vi "log analysis_gps.vi"() -> ()   [LabVIEW 2018] (continued)
-0.105000\n\t\n15:09:27.3\tlog_raw\tgps_raw\t#INSPVAXA,USB3,0,49.0,FINESTEERING,2107,281385.350,02000000,471d,15824;INS_ALIGNMENT_COMPLETE,INS_RTKFIXED,37.37092984687,126.72160192884,8.2009,22.3000,0.3659,0.2906,-0.0108,-0.966416737,-0.773960288,33.451430049,0.4185,0.2991,0.5729,0.1134,0.0948,0.0848,0.2660,0.2403,5.1498,0f000001,0*c2089fa9\n\tsystem status\tnormal 2 28.200000 0 0\trobot status\t67.923992\t88.748599\t8.200900\t-0.966417\t-0.773960\t56.548570\t0.472000\t0.029000\n\t\n15:09:27.8\tlog_raw\tgps_raw\t#INSPVAXA,USB3,0,49.0,FINESTEERING,2107,281385.850,02000000,471d,15824;INS_ALIGNMENT_COMPLETE,INS_RTKFIXED,37.37093156972,126.72160349245,8.1991,22.3000,0.3552,0.2819,0.0017,-0.982402524,-0.987093830,33.457221519,0.4185,0.2991,0.5729,0.1134,0.0948,0.0848,0.2660,0.2403,5.1498,0f000001,0*8db597c9\n\tsystem status\tnormal 2 28.200000 0 0\trobot status\t68.062494\t88.939808\t8.199100\t-0.982403\t-0.987094\t56.542778\t0.454000\t0.050000\n\t\n15:09:28.3\tlog_raw\tgps_raw\t\tsystem status\tnormal 2 28.200000 0 0\trobot status\t68.185778\t89.112120\t8.198400\t-0.951225\t-0.966912\t56.644351\t0.454000\t0.068000\n\t\n15:09:28.8\tlog_raw\tgps_raw\t#INSPVAXA,USB3,0,46.0,FINESTEERING,2107,281386.850,02000000,471d,15824;INS_ALIGNMENT_COMPLETE,INS_RTKFIXED,37.37093500656,126.72160657159,8.1978,22.3000,0.3860,0.2986,-0.0065,-0.930872832,-0.693352418,33.361120344,0.4182,0.2979,0.5715,0.1134,0.0948,0.0846,0.2660,0.2403,5.1494,0f000001,0*a8ec127a\n\tsystem status\tnormal 2 28.200000 0 0\trobot status\t68.335239\t89.321242\t8.197800\t-0.930873\t-0.693352\t56.638880\t0.495000\t0.011000\n\t\n15:09:29.3\tlog_raw\tgps_raw\t\tsystem status\tnormal 2 28.200000 0 0\trobot status\t68.463353\t89.496075\t8.196000\t-0.864589\t-0.927789\t56.656049\t0.556000\t-0.113000\n\t\n15:09:29.8\tlog_raw\tgps_raw\t#INSPVAXA,USB3,0,48.5,FINESTEERING,2107,281387.850,02000000,471d,15824;INS_ALIGNMENT_COMPLETE,INS_RTKFIXED,37.37093847805,126.72160977606,8.1934,22.3000,0.3545,0.2733,-0.0290,-0.871913936,-1.019858036,33.407520693,0.4181,0.2974,0.5707,0.1132,0.0948,0.0844,0.2660,0.2403,5.1492,0f000001,0*8b26d1b5\n\tsystem status\tnormal 2 28.200000 0 0\trobot status\t68.619086\t89.706522\t8.193400\t-0.871914\t-1.019858\t56.592479\t0.417000\t0.094000\n\t\n15:09:30.3\tlog_raw\tgps_raw\t\tsystem status\tnormal 2 28.200000 0 0\trobot status\t68.741379\t89.875198\t8.191600\t-0.846087\t-0.843708\t56.650263\t0.529000\t-0.019000\n\t\n15:09:30.8\tlog_raw\tgps_raw\t#INSPVAXA,USB3,0,47.0,FINESTEERING,2107,281388.850,02000000,471d,15824;INS_ALIGNMENT_COMPLETE,INS_RTKFIXED,37.37094185798,126.72161284652,8.1862,22.3000,0.3458,0.2807,0.0000,-0.647146834,-0.755815505,33.229882391,0.4177,0.2968,0.5693,0.1134,0.0951,0.0842,0.2659,0.2403,5.1493,0f000001,0*e04b9d7e\n\tsystem status\tnormal 2 28.200000 0 0\trobot status\t68.891062\t90.081640\t8.186200\t-0.647147\t-0.755816\t56.770118\t0.433000\t0.079000\n\t\n15:09:31.3\tlog_raw\tgps_raw\t\tsystem status\tnormal 2 28.200000 0 0\trobot status\t69.018551\t90.258982\t8.184300\t-0.770006\t-0.647307\t56.616583\t0.456000\t0.062000\n\t\n15:09:31.8\tlog_raw\tgps_raw\t#INSPVAXA,USB3,0,51.0,FINESTEERING,2107,281389.850,02000000,471d,15824;INS_ALIGNMENT_COMPLETE,INS_RTKFIXED,37.37094531152,126.72161597043,8.1814,22.3000,0.3770,0.3007,-0.0075,-0.964998734,-0.610692019,33.331132112,0.4178,0.2983,0.5697,0.1133,0.0955,0.0841,0.2659,0.2402,5.1491,0f000001,0*f3e7f4f6\n\tsystem status\tnormal 2 28.200000 0 0\trobot status\t69.167773\t90.464927\t8.181400\t-0.964999\t-0.610692\t56.668868\t0.457000\t0.069000\n\t\n15:09:32.3\tlog_raw\tgps_raw\t#INSPVAXA,USB3,0,50.5,FINESTEERING,2107,281390.350,02000000,471d,15824;INS_ALIGNMENT_COMPLETE,INS_RTKFIXED,37.37094699615,126.72161749721,8.1810,22.3000,0.3585,0.2781,-0.0176,-0.963426361,-0.735868518,33.269975778,0.4179,0.2987,0.5691,0.1132,0.0952,0.0837,0.2658,0.2402,5.1481,0f000001,0*d9e47fdc\n\tsystem status\tnormal 2 28.200000 0 0\trobot status\t69.303012\t90.651894\t8.181000\t-0.963426\t-0.735869\t56.730024\t0.431000\t0.076000\n\t\n15:09:32.8\tlog_raw\tgps_raw\t#INSPVAXA,USB3,0,50.5,FINESTEERING,2107,281390.850,02000000,471d,15824;INS_ALIGNMENT_COMPLETE,INS_RTKFIXED,37.37094874032,126.72161908849,8.1805,22.3000,0.3294,0.2293,-0.0009,-0.908401670,-0.595727338,33.364278854,0.4179,0.2987,0.5691,0.1132,0.0952,0.0837,0.2658,0.2402,5.1481,0f000001,0*5999a9d2\n\tsystem status\tnormal 2 28.200000 0 0\trobot status\t69.443965\t90.845469\t8.180500\t-0.908402\t-0.595727\t56.635721\t0.644000\t-0.257000\n\t\n15:09:33.3\tlog_raw\tgps_raw\t#INSPVAXA,USB3,0,48.0,FINESTEERING,2107,281391.350,02000000,471d,15824;INS_ALIGNMENT_COMPLETE,INS_RTKFIXED,37.37095049924,126.72162069173,8.1796,22.3000,0.4034,0.3085,-0.0112,-0.795383493,-0.971346032,33.378242699,0.4182,0.2986,0.5686,0.1132,0.0949,0.0836,0.2658,0.2402,5.1464,0f000001,0*1e48eff8\n\tsystem status\tnormal 2 28.200000 0 0\trobot status\t69.585978\t91.040681\t8.179600\t-0.795383\t-0.971346\t56.621757\t0.521000\t-0.011000\n\t\n15:09:33.8\tlog_raw\tgps_raw\t#INSPVAXA,USB3,0,48.0,FINESTEERING,2107,281391.850,02000000,471d,15824;INS_ALIGNMENT_COMPLETE,INS_RTKFIXED,37.37095218768,126.72162223158,8.1782,22.3000,0.3736,0.3039,0.0085,-0.869440972,-1.042554722,33.323263236,0.4182,0.2986,0.5686,0.1132,0.0949,0.0836,0.2658,0.2402,5.1464,0f000001,0*be662b3c\n\tsystem status\tnormal 2 28.200000 0 0\trobot status\t69.722375\t91.228070\t8.178200\t-0.869441\t-1.042555\t56.676737\t0.524000\t-0.028000\n\t\n15:09:34.3\tlog_raw\tgps_raw\t\tsystem status\tnormal 2 28.200000 0 0\trobot status\t69.851097\t91.401055\t8.175700\t-0.533369\t-1.495352\t56.519855\t0.436000\t0.040000\n\t\n15:09:34.8\tlog_raw\tgps_raw\t#INSPVAXA,USB3,0,46.5,FINESTEERING,2107,281392.850,02000000,471d,15824;INS_ALIGNMENT_COMPLETE,INS_RTKFIXED,37.37095563956,126.72162543709,8.1738,22.3000,0.3750,0.2874,-0.0042,-0.381103782,-1.196591916,33.536451772,0.4182,0.2976,0.5666,0.1131,0.0944,0.0833,0.2657,0.2401,5.1446,0f000001,0*fd2c5164\n\tsystem status\tnormal 2 28.200000 0 0\trobot status\t70.006314\t91.611174\t8.173800\t-0.381104\t-1.196592\t56.463548\t0.516000\t-0.027000\n\t\n15:09:35.3\tlog_raw\tgps_raw\t#INSPVAXA,USB3,0,47.0,FINESTEERING,2107,281393.350,02000000,471d,15824;INS_ALIGNMENT_COMPLETE,INS_RTKFIXED,37.37095732903,126.72162695963,8.1710,22.3000,0.3684,0.2951,-0.0131,-0.615904330,-1.127921907,33.544859726,0.4171,0.2952,0.5633,0.1132,0.0946,0.0833,0.2656,0.2401,5.1445,0f000001,0*dbe231da\n\tsystem status\tnormal 2 28.200000 0 0\trobot status\t70.141178\t91.798678\t8.171000\t-0.615904\t-1.127922\t56.455140\t0.493000\t0.009000\n\t\n15:09:35.8\tlog_raw\tgps_raw\t#INSPVAXA,USB3,0,47.0,FINESTEERING,2107,281393.850,02000000,471d,15824;INS_ALIGNMENT_COMPLETE,INS_RTKFIXED,37.37095908537,126.72162857603,8.1657,22.3000,0.3533,0.2801,-0.0216,-0.431209048,-1.265989093,33.662345403,0.4171,0.2952,0.5633,0.1132,0.0946,0.0833,0.2656,0.2401,5.1445,0f000001,0*22a3a0dc\n\tsystem status\tnormal 2 28.200000 0 0\trobot status\t70.284356\t91.993603\t8.165700\t-0.431209\t-1.265989\t56.337655\t0.473000\t0.013000\n\t\n15:09:36.3\tlog_raw\tgps_raw\t#INSPVAXA,USB3,0,49.5,FINESTEERING,2107,281394.350,02000000,471d,15824;INS_ALIGNMENT_COMPLETE,INS_RTKFIXED,37.37096076368,126.72163015176,8.1608,22.3000,0.3647,0.2816,-0.0115,-0.296506050,-1.118124475,33.712011853,0.4164,0.2937,0.5589,0.1136,0.0946,0.0836,0.2655,0.2400,5.1444,0f000001,0*688a566e\n\tsystem status\tnormal 2 28.200000 0 0\trobot status\t70.423932\t92.179869\t8.160800\t-0.296506\t-1.118124\t56.287988\t0.497000\t0.000000\n\t\n15:09:36.8\tlog_raw\tgps_raw\t#INSPVAXA,USB3,0,49.5,FINESTEERING,2107,281394.850,02000000,471d,15824;INS_ALIGNMENT_COMPLETE,INS_RTKFIXED,37.37096245961,126.72163173093,8.1552,22.3000,0.3611,0.2897,0.0065,-0.395039042,-1.114938757,33.806057490,0.4164,0.2937,0.5589,0.1136,0.0946,0.0836,0.2655,0.2400,5.1444,0f000001,0*207a4651\n\tsystem status\tnormal 2 28.200000 0 0\trobot status\t70.563812\t92.368089\t8.155200\t-0.395039\t-1.114939\t56.193943\t0.482000\t0.013000\n\t\n15:09:37.3\tlog_raw\tgps_raw\t\tsystem status\tnormal 2 28.200000 0 0\trobot status\t70.685779\t92.532461\t8.150200\t-0.328345\t-0.854593\t56.176913\t0.501000\t-0.012000\n\t\n15:09:37.8\tlog_raw\tgps_raw\t#INSPVAXA,USB3,0,47.5,FINESTEERING,2107,281395.850,02000000,471d,15824;INS_ALIGNMENT_COMPLETE,INS_RTKFIXED,37.37096587417,126.72163486610,8.1446,22.3000,0.3698,0.2924,-0.0143,-0.371056293,-0.946940262,33.969984358,0.4152,0.2922,0.5549,0.1139,0.0950,0.0842,0.2655,0.2400,5.1444,0f000001,0*416a3ff6\n\tsystem status\tnormal 2 28.200000 0 0\trobot status\t70.841520\t92.747051\t8.144600\t-0.371056\t-0.946940\t56.030016\t0.509000\t-0.014000\n\t\n15:09:38.3\tlog_raw\tgps_raw\t#INSPVAXA,USB3,0,47.5,FINESTEERING,2107,281396.350,02000000,471d,15824;INS_ALIGNMENT_COMPLETE,INS_RTKFIXED,37.37096753829,126.72163640742,8.1378,22.3000,0.3398,0.2681,-0.0087,-0.164596770,-1.133388969,33.930144164,0.4145,0.2919,0.5524,0.1132,0.0937,0.0831,0.2654,0.2399,5.1441,0f000001,0*c9e3845c\n\tsystem status\tnormal 2 28.200000 0 0\trobot status\t70.978048\t92.931741\t8.137800\t-0.164597\t-1.133389\t56.069856\t0.415000\t0.100000\n\t\n15:09:38.8\tlog_raw\tgps_raw\t#INSPVAXA,USB3,0,47.5,FINESTEERING,2107,281396.850,02000000,471d,15824;INS_ALIGNMENT_COMPLETE,INS_RTKFIXED,37.37096924651,126.72163797428,8.1309,22.3000,0.3574,0.2705,-0.0020,-0.147004218,-0.814443066,33.921255816,0.4145,0.2919,0.5524,0.1132,0.0937,0.0831,0.2654,0.2399,5.1441,0f000001,0*98005433\n\tsystem status\tnormal 2 28.200000 0 0\trobot status\t71.116838\t93.121326\t8.130900\t-0.147004\t-0.814443\t56.078744\t0.431000\t0.089000\n\t\n15:09:39.3\tlog_raw\tgps_raw\t#INSPVAXA,USB3,0,49.5,FINESTEERING,2107,281397.350,02000000,471d,15824;INS_ALIGNMENT_COMPLETE,INS_RTKFIXED,37.37097094637,126.72163952751,8.1230,22.3000,0.3568,0.2763,-0.0303,-0.204424116,-0.677389898,33.930384401,0.4166,0.2976,0.5621,0.1134,0.0950,0.0840,0.2655,0.2398,5.1447,0f000001,0*229e290a\n\tsystem status\tnormal 2 28.200000 0 0\trobot status\t71.254420\t93.309983\t8.123000\t-0.204424\t-0.677390\t56.069616\t0.437000\t0.088000\n\t\n15:09:39.8\tlog_raw\tgps_raw\t#INSPVAXA,USB3,0,49.5,FINESTEERING,2107,281397.850,02000000,471d,15824;INS_ALIGNMENT_COMPLETE,INS_RTKFIXED,37.37097267317,126.72164110503,8.1156,22.3000,0.3644,0.2601,0.0030,-0.207601893,-0.850493393,33.903346021,0.4166,0.2976,0.5621,0.1134,0.0950,0.0840,0.2655,0.2398,5.1447,0f000001,0*99e15a33\n\tsystem status\tnormal 2 28.200000 0 0\trobot status\t71.394154\t93.501630\t8.115600\t-0.207602\t-0.850493\t56.096654\t0.434000\t0.077000\n\t\n15:09:40.3\tlog_raw\tgps_raw\t#INSPVAXA,USB3,0,47.0,FINESTEERING,2107,281398.350,02000000,471d,15824;INS_ALIGNMENT_COMPLETE,INS_RTKFIXED,37.37097438871,126.72164266550,8.1100,22.3000,0.3561,0.2764,-0.0101,-0.236656715,-0.969278432,33.883238770,0.4175,0.2995,0.5669,0.1134,0.0951,0.0842,0.2654,0.2398,5.1455,0f000001,0*71e938c6\n\tsystem status\tnormal 2 28.200000 0 0\trobot status\t71.532378\t93.692028\t8.110000\t-0.236657\t-0.969278\t56.116761\t0.440000\t0.086000\n\t\n15:09:40.8\tlog_raw\tgps_raw\t#INSPVAXA,USB3,0,47.0,FINESTEERING,2107,281398.850,02000000,471d,15824;INS_ALIGNMENT_COMPLETE,INS_RTKFIXED,37.37097610679,126.72164421082,8.1028,22.3000,0.3606,0.2818,-0.0239,-0.382752172,-0.849124601,34.007737280,0.4175,0.2995,0.5669,0.1134,0.0951,0.0842,0.2654,0.2398,5.1455,0f000001,0*8bea9a1b\n\tsystem status\tnormal 2 28.200000 0 0\trobot status\t71.669260\t93.882707\t8.102800\t-0.382752\t-0.849125\t55.992263\t0.544000\t-0.080000\n\t\n15:09:41.3\tlog_raw\tgps_raw\t#INSPVAXA,USB3,0,48.0,FINESTEERING,2107,281399.350,02000000,471d,15824;INS_ALIGNMENT_COMPLETE,INS_RTKFIXED,37.37097781437,126.72164579637,8.0962,22.3000,0.3464,0.2856,-0.0229,-0.220443352,-0.638082090,34.139023670,0.4187,0.3008,0.5721,0.1133,0.0950,0.0843,0.2654,0.2397,5.1467,0f000001,0*4de46431\n\tsystem status\tnormal 2 28.200000 0 0\trobot status\t71.809706\t94.072221\t8.096200\t-0.220443\t-0.638082\t55.860976\t0.490000\t-0.003000\n\t\n15:09:41.8\tlog_raw\tgps_raw\t#INSPVAXA,USB3,0,48.0,FINESTEERING,2107,281399.850,02000000,471d,15824;INS_ALIGNMENT_COMPLETE,INS_RTKFIXED,37.37097954920,126.72164741016,8.0894,22.3000,0.3776,0.2848,-0.0077,-0.220802619,-0.919793940,34.236212275,0.4187,0.3008,0.5721,0.1133,0.0950,0.0843,0.2654,0.2397,5.1467,0f000001,0*1294b3ed\n\tsystem status\tnormal 2 28.200000 0 0\trobot status\t71.952652\t94.264759\t8.089400\t-0.220803\t-0.919794\t55.763788\t0.496000\t-0.003000\n\t\n15:09:42.3\tlog_raw\tgps_raw\t#INSPVAXA,USB3,0,51.0,FINESTEERING,2107,281400.350,02000000,471d,15824;INS_ALIGNMENT_COMPLETE,INS_RTKFIXED,37.37098127121,126.72164900828,8.0835,22.3000,0.3512,0.2798,-0.0167,-0.348314510,-1.071908763,34.359634607,0.4200,0.3034,0.5796,0.1133,0.0952,0.0845,0.2654,0.2397,5.1479,0f000001,0*0d7d68ff\n\tsystem status\tnormal 2 28.200000 0 0\trobot status\t72.094211\t94.455874\t8.083500\t-0.348315\t-1.071909\t55.640365\t0.488000\t0.004000\n\t\n15:09:42.8\tlog_raw\tgps_raw\t\tsystem status\tnormal 2 28.200000 0 0\trobot status\t72.235639\t94.643836\t8.077100\t-0.443262\t-0.875036\t55.562836\t0.488000\t0.000000\n\t\n15:09:43.3\tlog_raw\tgps_raw\t#INSPVAXA,USB3,0,47.5,FINESTEERING,2107,281401.350,02000000,471d,15824;INS_ALIGNMENT_COMPLETE,INS_RTKFIXED,37.37098468255,126.72165224111,8.0693,22.3000,0.3522,0.2654,-0.0166,-0.377347631,-0.696818935,34.675390534,0.4199,0.3031,0.5827,0.1133,0.0950,0.0845,0.2653,0.2397,5.1493,0f000001,0*9d8e74ce\n\tsystem status\tnormal 2 28.200000 0 0\trobot status\t72.380570\t94.834478\t8.069300\t-0.377348\t-0.696819\t55.324609\t0.489000\t-0.012000\n\t\n15:09:43.8\tlog_raw\tgps_raw\t#INSPVAXA,USB3,0,47.5,FINESTEERING,2107,281401.850,02000000,471d,15824;INS_ALIGNMENT_COMPLETE,INS_RTKFIXED,37.37098640066,126.72165387594,8.0604,22.3000,0.3637,0.3053,-0.0327,-0.270135271,-0.804168366,34.795363793,0.4199,0.3031,0.5827,0.1133,0.0950,0.0845,0.2653,0.2397,5.1493,0f000001,0*da64b754\n\tsystem status\tnormal 2 28.200000 0 0\trobot status\t72.525381\t95.025161\t8.060400\t-0.270135\t-0.804168\t55.204636\t0.506000\t-0.006000\n\t\n15:09:44.3\tlog_raw\tgps_raw\t#INSPVAXA,USB3,0,50.5,FINESTEERING,2107,281402.350,02000000,471d,15824;INS_ALIGNMENT_COMPLETE,INS_RTKFIXED,37.37098814311,126.72165553313,8.0529,22.3000,0.3514,0.2761,-0.0227,-0.415994366,-1.222362731,34.800018159,0.4207,0.3056,0.5893,0.1133,0.0953,0.0846,0.2653,0.2396,5.1507,0f000001,0*f3097738\n\tsystem status\tnormal 2 28.200000 0 0\trobot status\t72.672172\t95.218545\t8.052900\t-0.415994\t-1.222363\t55.199982\t0.505000\t-0.016000\n\t\n15:09:44.8\tlog_raw\tgps_raw\t#INSPVAXA,USB3,0,50.5,FINESTEERING,2107,281402.850,02000000,471d,15824;INS_ALIGNMENT_COMPLETE,INS_RTKFIXED,37.37098982425,126.72165714706,8.0452,22.3000,0.3664,0.2820,-0.0237,-0.514294339,-1.108715950,34.873142980,0.4207,0.3056,0.5893,0.1133,0.0953,0.0846,0.2653,0.2396,5.1507,0f000001,0*3533bd5f\n\tsystem status\tnormal 2 28.200000 0 0\trobot status\t72.815131\t95.405124\t8.045200\t-0.514294\t-1.108716\t55.126857\t0.489000\t0.035000\n\t\n15:09:45.3\tlog_raw\tgps_raw\t#INSPVAXA,USB3,0,46.5,FINESTEERING,2107,281403.350,02000000,471d,15824;INS_ALIGNMENT_COMPLETE,INS_RTKFIXED,37.37099150836,126.72165880250,8.0350,22.3000,0.3619,0.2923,-0.0388,-0.135694474,-1.036034406,34.888546976,0.4207,0.3066,0.5937,0.1132,0.0955,0.0846,0.2653,0.2396,5.1519,0f000001,0*7db2ed89\n\tsystem status\tnormal 2 28.200000 0 0\trobot status\t72.961767\t95.592033\t8.035000\t-0.135694\t-1.036034\t55.111453\t0.474000\t0.035000\n\t\n15:09:45.8\tlog_raw\tgps_raw\t\tsystem status\tnormal 2 28.200000 0 0\trobot status\t73.108224\t95.779809\t8.025900\t-0.239720\t-1.094114\t55.107036\t0.426000\t0.086000\n\t\n15:09:46.3\tlog_raw\tgps_raw\t#INSPVAXA,USB3,0,45.5,FINESTEERING,2107,281404.350,02000000,471d,15824;INS_ALIGNMENT_COMPLETE,INS_RTKFIXED,37.37099493279,126.72166212564,8.0179,22.3000,0.3493,0.2735,-0.0199,-0.409952245,-1.106661495,34.971995764,0.4183,0.3008,0.5856,0.1131,0.0947,0.0839,0.2651,0.2395,5.1529,0f000001,0*541bafca\n\tsystem status\tnormal 2 28.200000 0 0\trobot status\t73.256126\t95.972089\t8.017900\t-0.409952\t-1.106661\t55.028004\t0.420000\t0.106000\n\t\n15:09:46.8\tlog_raw\tgps_raw\t#INSPVAXA,USB3,0,45.5,FINESTEERING,2107,281404.850,02000000,471d,15824;INS_ALIGNMENT_COMPLETE,INS_RTKFIXED,37.37099660227,126.72166374929,8.0125,22.3000,0.3621,0.2956,-0.0286,-0.267167833,-0.753528343,34.912800683,0.4183,0.3008,0.5856,0.1131,0.0947,0.0839,0.2651,0.2395,5.1529,0f000001,0*d35c1563\n\tsystem status\tnormal 2 28.200000 0 0\trobot status\t73.399946\t96.157375\t8.012500\t-0.267168\t-0.753528\t55.087199\t0.470000\t0.039000\n\t\n15:09:47.3\tlog_raw\tgps_raw\t#INSPVAXA,USB3,0,47.0,FINESTEERING,2107,281405.350,02000000,471d,15824;INS_ALIGNMENT_COMPLETE,INS_RTKFIXED,37.37099831104,126.72166542304,8.0059,22.3000,0.3575,0.2905,-0.0163,-0.253871476,-0.573976572,34.788811837,0.4180,0.3006,0.5851,0.1139,0.0957,0.0850,0.2651,0.2394,5.1534,0f000001,0*ea0daca7\n\tsystem status\tnormal 2 28.200000 0 0\trobot status\t73.548204\t96.347021\t8.005900\t-0.253871\t-0.573977\t55.211188\t0.601000\t-0.155000\n\t\n15:09:47.8\tlog_raw\tgps_raw\t#INSPVAXA,USB3,0,47.0,FINESTEERING,2107,281405.850,02000000,471d,15824;INS_ALIGNMENT_COMPLETE,INS_RTKFIXED,37.37100000968,126.72166711041,8.0001,22.3000,0.3748,0.2860,-0.0242,-0.088360721,-0.852531468,34.685538696,0.4180,0.3006,0.5851,0.1139,0.0957,0.0850,0.2651,0.2394,5.1534,0f000001,0*79314379\n\tsystem status\tnormal 2 28.200000 0 0\trobot status\t73.697668\t96.535542\t8.000100\t-0.088361\t-0.852531\t55.314461\t0.436000\t0.085000\n\t\n15:09:48.3\tlog_raw\tgps_raw\t#INSPVAXA,USB3,0,49.0,FINESTEERING,2107,281406.350,02000000,471d,15824;INS_ALIGNMENT_COMPLETE,INS_RTKFIXED,37.37100175880,126.72166880875,7.9944,22.3000,0.3745,0.2914,-0.0180,-0.078489468,-1.009185003,34.665355987,0.4165,0.2969,0.5768,0.1147,0.0961,0.0860,0.2650,0.2394,5.1543,0f000001,0*41bb7608\n\tsystem status\tnormal 2 28.200000 0 0\trobot status\t73.848104\t96.729666\t7.994400\t-0.078489\t-1.009185\t55.334644\t0.601000\t-0.154000\n\t\n15:09:48.8\tlog_raw\tgps_raw\t\tsystem status\tnormal 2 28.200000 0 0\trobot status\t73.990114\t96.914205\t7.989900\t-0.212224\t-1.085393\t55.584584\t0.585000\t-0.126000\n\t\n15:09:49.3\tlog_raw\tgps_raw\t#INSPVAXA,USB3,0,49.0,FINESTEERING,2107,281407.350,02000000,471d,15824;INS_ALIGNMENT_COMPLETE,INS_RTKFIXED,37.37100512322,126.72167206883,7.9829,22.3000,0.3677,0.2809,-0.0383,0.055269502,-0.871990606,34.333614581,0.4159,0.2956,0.5723,0.1160,0.0974,0.0881,0.2649,0.2393,5.1550,0f000001,0*e297d913\n\tsystem status\tnormal 2 28.200000 0 0\trobot status\t74.136877\t97.103063\t7.982900\t0.055270\t-0.871991\t55.666385\t0.443000\t0.053000\n\t\n15:09:49.8\tlog_raw\tgps_raw\t#INSPVAXA,USB3,0,49.0,FINESTEERING,2107,281407.850,02000000,471d,15824;INS_ALIGNMENT_COMPLETE,INS_RTKFIXED,37.37100682475,126.72167368991,7.9758,22.3000,0.3450,0.2906,-0.0278,0.076806319,-0.668802116,34.237004586,0.4159,0.2956,0.5723,0.1160,0.0974,0.0881,0.2649,0.2393,5.1550,0f000001,0*eb42bcbe\n\tsystem status\tnormal 2 28.200000 0 0\trobot status\t74.280470\t97.291905\t7.975800\t0.076806\t-0.668802\t55.762995\t0.604000\t-0.162000\n\t\n15:09:50.3\tlog_raw\tgps_raw\t#INSPVAXA,USB3,0,49.0,FINESTEERING,2107,281408.350,02000000,471d,15824;INS_ALIGNMENT_COMPLETE,INS_RTKFIXED,37.37100857076,126.72167534247,7.9736,22.3000,0.3634,0.2846,-0.0190,-0.182813493,-0.879750967,34.094650062,0.4161,0.2965,0.5711,0.1145,0.0958,0.0868,0.2649,0.2393,5.1559,0f000001,0*ba1fbbd1\n\tsystem status\tnormal 2 28.200000 0 0\trobot status\t74.426851\t97.485684\t7.973600\t-0.182813\t-0.879751\t55.905350\t0.442000\t0.069000\n\t\n15:09:50.8\tlog_raw\tgps_raw\t#INSPVAXA,USB3,0,49.0,FINESTEERING,2107,281408.850,02000000,471d,15824;INS_ALIGNMENT_COMPLETE,INS_RTKFIXED,37.37101026525,126.72167697337,7.9727,22.3000,0.3524,0.2783,-0.0246,-0.098737305,-0.690752334,33.910631500,0.4161,0.2965,0.5711,0.1145,0.0958,0.0868,0.2649,0.2393,5.1559,0f000001,0*d5b16fe8\n\tsystem status\tnormal 2 28.200000 0 0\trobot status\t74.571313\t97.673745\t7.972700\t-0.098737\t-0.690752\t56.089368\t0.575000\t-0.126000\n\t\n15:09:51.3\tlog_raw\tgps_raw\t#INSPVAXA,USB3,0,47.5,FINESTEERING,2107,281409.350,02000000,471d,15824;INS_ALIGNMENT_COMPLETE,INS_RTKFIXED,37.37101200437,126.72167857017,7.9719,22.3000,0.3673,0.3066,-0.0244,-0.420788016,-0.858221661,33.836234761,0.4162,0.2973,0.5715,0.1138,0.0952,0.0865,0.2649,0.2392,5.1570,0f000001,0*5513fa8f\n\tsystem status\tnormal 2 28.200000 0 0\trobot status\t74.712755\t97.866759\t7.971900\t-0.420788\t-0.858222\t56.163765\t0.434000\t0.095000\n\t\n15:09:51.8\tlog_raw\tgps_raw\t\tsystem status\tnormal 2 28.200000 0 0\trobot status\t74.852613\t98.053840\t7.974800\t-0.237218\t-0.495171\t56.233078\t0.575000\t-0.126000\n\t\n15:09:52.3\tlog_raw\tgps_raw\t\tsystem status\tnormal 2 28.200000 0 0\trobot status\t74.996403\t98.249011\t7.971900\t-0.241180\t-0.783626\t56.276468\t0.493000\t0.017000\n\t\n15:09:52.8\tlog_raw\tgps_raw\t#INSPVAXA,USB3,0,49.0,FINESTEERING,2107,281410.850,02000000,471d,15824;INS_ALIGNMENT_COMPLETE,INS_RTKFIXED,37.37101714160,126.72168333239,7.9694,22.3000,0.3574,0.2819,-0.0127,-0.504237932,-0.910801054,33.584207367,0.4157,0.2969,0.5709,0.1135,0.0948,0.0862,0.2649,0.2392,5.1584,0f000001,0*1e770ccd\n\tsystem status\tnormal 2 28.200000 0 0\trobot status\t75.134585\t98.436909\t7.969400\t-0.504238\t-0.910801\t56.415793\t0.444000\t0.063000\n\t\n15:09:53.3\tlog_raw\tgps_raw\t#INSPVAXA,USB3,0,49.0,FINESTEERING,2107,281411.350,02000000,471d,15824;INS_ALIGNMENT_COMPLETE,INS_RTKFIXED,37.37101885346,126.72168493250,7.9707,22.3000,0.3563,0.2832,-0.0055,-0.267715843,-0.919384787,33.461951362,0.4158,0.2973,0.5713,0.1134,0.0948,0.0862,0.2649,0.2392,5.1601,0f000001,0*2f0cc835\n\tsystem status\tnormal 2 28.200000 0 0\trobot status\t75.276320\t98.626898\t7.970700\t-0.267716\t-0.919385\t56.538049\t0.459000\t0.055000\n\t\n15:09:53.8\tlog_raw\tgps_raw\t#INSPVAXA,USB3,0,49.0,FINESTEERING,2107,281411.850,02000000,471d,15824;INS_ALIGNMENT_COMPLETE,INS_RTKFIXED,37.37102056914,126.72168651879,7.9675,22.3000,0.3602,0.2584,-0.0273,-0.124586841,-0.381382122,33.473261992,0.4158,0.2973,0.5713,0.1134,0.0948,0.0862,0.2649,0.2392,5.1601,0f000001,0*eba26ee8\n\tsystem status\tnormal 2 28.200000 0 0\trobot status\t75.416831\t98.817311\t7.967500\t-0.124587\t-0.381382\t56.526738\t0.447000\t0.063000\n\t\n15:09:54.3\tlog_raw\tgps_raw\t\tsystem status\tnormal 2 28.200000 0 0\trobot status\t75.553164\t99.007976\t7.967400\t-0.401644\t-0.367575\t56.596971\t0.499000\t0.009000\n\t\n15:09:54.8\tlog_raw\tgps_raw\t#INSPVAXA,USB3,0,50.5,FINESTEERING,2107,281412.850,02000000,471d,15824;INS_ALIGNMENT_COMPLETE,INS_RTKFIXED,37.37102404142,126.72168963423,7.9673,22.3000,0.3604,0.2695,-0.0148,-0.373966632,-0.606948860,33.415990980,0.4147,0.2955,0.5683,0.1128,0.0939,0.0847,0.2648,0.2392,5.1618,0f000001,0*2af052bc\n\tsystem status\tnormal 2 28.200000 0 0\trobot status\t75.692791\t99.202678\t7.967300\t-0.373967\t-0.606949\t56.584009\t0.552000\t-0.120000\n\t\n15:09:55.3\tlog_raw\tgps_raw\t\tsystem status\tnormal 2 28.200000 0 0\trobot status\t75.831473\t99.394247\t7.966600\t-0.273773\t-0.729126\t56.599673\t0.473000\t0.036000\n\t\n15:09:55.8\tlog_raw\tgps_raw\t#INSPVAXA,USB3,0,50.0,FINESTEERING,2107,281413.850,02000000,471d,15824;INS_ALIGNMENT_COMPLETE,INS_RTKFIXED,37.37102747823,126.72169275298,7.9678,22.3000,0.3771,0.2870,-0.0120,-0.268357218,-0.590747606,33.358928926,0.4139,0.2944,0.5647,0.1119,0.0930,0.0833,0.2648,0.2392,5.1630,0f000001,0*49d73869\n\tsystem status\tnormal 2 28.200000 0 0\trobot status\t75.969045\t99.584108\t7.967800\t-0.268357\t-0.590748\t56.641071\t0.512000\t-0.013000\n\t\n15:09:56.3\tlog_raw\tgps_raw\t#INSPVAXA,USB3,0,52.0,FINESTEERING,2107,281414.350,02000000,471d,15824;INS_ALIGNMENT_COMPLETE,INS_RTKFIXED,37.37102919906,126.72169428812,7.9675,22.3000,0.3604,0.2661,-0.0032,-0.659688126,-0.428969393,33.411905662,0.4132,0.2936,0.5618,0.1122,0.0937,0.0832,0.2648,0.2392,5.1641,0f000001,0*c98d060a\n\tsystem status\tnormal 2 28.200000 0 0\trobot status\t76.105025\t99.775093\t7.967500\t-0.659688\t-0.428969\t56.588094\t0.556000\t-0.100000\n\t\n15:09:56.8\tlog_raw\tgps_raw\t\tsystem status\tnormal 2 28.200000 0 0\trobot status\t76.244276\t99.968310\t7.967300\t-0.494857\t-0.442528\t56.570833\t0.518000\t-0.036000\n\t\n15:09:57.3\tlog_raw\tgps_raw\t#INSPVAXA,USB3,0,44.5,FINESTEERING,2107,281415.350,02000000,471d,15824;INS_ALIGNMENT_COMPLETE,INS_RTKFIXED,37.37103267995,126.72169744869,7.9665,22.3000,0.3768,0.2993,-0.0116,-0.528478591,-0.759705931,33.438134045,0.4126,0.2929,0.5591,0.1118,0.0933,0.0820,0.2647,0.2392,5.1652,0f000001,0*581dc28c\n\tsystem status\tnormal 2 28.200000 0 0\trobot status\t76.384983\t100.161415\t7.966500\t-0.528479\t-0.759706\t56.561866\t0.488000\t0.014000\n\t\n15:09:57.8\tlog_raw\tgps_raw\t\tsystem status\tnormal 2 28.200000 0 0\trobot status\t76.527285\t100.354860\t7.964400\t-0.649744\t-0.685748\t56.395095\t0.416000\t0.092000\n\t\n15:09:58.3\tlog_raw\tgps_raw\t#INSPVAXA,USB3,0,48.5,FINESTEERING,2107,281416.350,02000000,471d,15824;INS_ALIGNMENT_COMPLETE,INS_RTKFIXED,37.37103613052,126.72170062414,7.9635,22.3000,0.4087,0.2756,-0.0246,-0.725160800,-0.633419776,33.720037993,0.4128,0.2920,0.5564,0.1119,0.0930,0.0810,0.2647,0.2392,5.1665,0f000001,0*1631f0a5\n\tsystem status\tnormal 2 28.200000 0 0\trobot status\t76.666260\t100.544373\t7.963500\t-0.725161\t-0.633420\t56.279962\t0.524000\t-0.032000\n\t\n15:09:58.8\tlog_raw\tgps_raw\t\tsystem status\tnormal 2 28.200000 0 0\trobot status\t76.809704\t100.736116\t7.962200\t-0.593733\t-0.742817\t56.249227\t0.480000\t0.009000\n\t\n15:09:59.3\tlog_raw\tgps_raw\t#INSPVAXA,USB3,0,48.5,FINESTEERING,2107,281417.350,02000000,471d,15824;INS_ALIGNMENT_COMPLETE,INS_RTKFIXED,37.37103952444,126.72170377706,7.9632,22.3000,0.3570,0.2779,-0.0018,-0.570124026,-0.772949889,33.647986362,0.4118,0.2899,0.5509,0.1122,0.0932,0.0810,0.2645,0.2391,5.1675,0f000001,0*233b5573\n\tsystem status\tnormal 2 28.200000 0 0\trobot status\t76.945540\t100.921043\t7.963200\t-0.570124\t-0.772950\t56.352014\t0.440000\t0.077000\n\t\n15:09:59.8\tlog_raw\tgps_raw\t#INSPVAXA,USB3,0,48.5,FINESTEERING,2107,281417.850,02000000,471d,15824;INS_ALIGNMENT_COMPLETE,INS_RTKFIXED,37.37104128675,126.72170534574,7.9659,22.3000,0.3708,0.2756,-0.0283,-0.789006262,-0.544112673,33.784716774,0.4118,0.2899,0.5509,0.1122,0.0932,0.0810,0.2645,0.2391,5.1675,0f000001,0*dc8c1e25\n\tsystem status\tnormal 2 28.200000 0 0\trobot status\t77.084491\t101.116631\t7.965900\t-0.789006\t-0.544113\t56.215283\t0.441000\t0.097000\n\t\n15:10:00.3\tlog_raw\tgps_raw\t\tsystem status\tnormal 2 28.200000 0 0\trobot status\t77.222413\t101.303872\t7.964300\t-0.716340\t-0.699945\t56.254621\t0.512000\t-0.015000\n\t\n15:10:00.8\tlog_raw\tgps_raw\t#INSPVAXA,USB3,0,49.0,FINESTEERING,2107,281418.850,02000000,471d,15824;INS_ALIGNMENT_COMPLETE,INS_RTKFIXED,37.37104464340,126.72170847296,7.9663,22.3000,0.3685,0.2500,0.0007,-0.664002073,-0.601650927,33.708955665,0.4113,0.2892,0.5478,0.1120,0.0929,0.0802,0.2644,0.2390,5.1688,0f000001,0*3627658d\n\tsystem status\tnormal 2 28.200000 0 0\trobot status\t77.361495\t101.489165\t7.966300\t-0.664002\t-0.601651\t56.291044\t0.523000\t-0.065000\n\t\n15:10:01.3\tlog_raw\tgps_raw\t\tsystem status\tnormal 2 28.200000 0 0\trobot status\t77.505596\t101.685079\t7.966100\t-0.757035\t-0.904575\t56.276935\t0.573000\t-0.127000\n\t\n15:10:01.8\tlog_raw\tgps_raw\t\tsystem status\tnormal 2 28.200000 0 0\trobot status\t77.644718\t101.868896\t7.966900\t-0.488055\t-0.475273\t56.343535\t0.577000\t-0.120000\n\t\n15:10:02.3\tlog_raw\tgps_raw\t#INSPVAXA,USB3,0,49.5,FINESTEERING,2107,281420.350,02000000,471d,15824;INS_ALIGNMENT_COMPLETE,INS_RTKFIXED,37.37104977182,126.72171326330,7.9681,22.3000,0.3654,0.2752,-0.0075,-0.486218413,-0.454617535,33.615388991,0.4147,0.2981,0.5609,0.1124,0.0945,0.0810,0.2643,0.2389,5.1711,0f000001,0*c1b15c55\n\tsystem status\tnormal 2 28.200000 0 0\trobot status\t77.785816\t102.058337\t7.968100\t-0.486218\t-0.454618\t56.384611\t0.585000\t-0.124000\n\t\n15:10:02.8\tlog_raw\tgps_raw\t\tsystem status\tnormal 2 28.200000 0 0\trobot status\t77.928673\t102.247731\t7.967200\t-0.199654\t-0.312772\t56.474939\t0.485000\t0.030000\n\t\n15:10:03.3\tlog_raw\tgps_raw\t\tsystem status\tnormal 2 28.200000 0 0\trobot status\t78.070590\t102.436178\t7.969000\t-0.151885\t-0.672761\t56.576914\t0.467000\t0.033000\n\t\n15:10:03.8\tlog_raw\tgps_raw\t#INSPVAXA,USB3,0,49.0,FINESTEERING,2107,281421.850,02000000,471d,15824;INS_ALIGNMENT_COMPLETE,INS_RTKFIXED,37.37105483304,126.72171804762,7.9714,22.3000,0.3720,0.2729,0.0059,-0.226869294,-0.357217167,33.322901739,0.4153,0.3006,0.5651,0.1122,0.0940,0.0806,0.2643,0.2388,5.1727,0f000001,0*c9d844c6\n\tsystem status\tnormal 2 28.200000 0 0\trobot status\t78.209603\t102.620050\t7.971400\t-0.226869\t-0.357217\t56.677098\t0.587000\t-0.126000\n\t\n15:10:04.3\tlog_raw\tgps_raw\t\tsystem status\tnormal 2 28.200000 0 0\trobot status\t78.349385\t102.808247\t7.971300\t-0.248573\t0.003587\t56.717206\t0.467000\t0.036000\n\t\n15:10:04.8\tlog_raw\tgps_raw\t\tsystem status\tnormal 2 28.200000 0 0\trobot status\t78.490333\t102.997185\t7.972000\t-0.114687\t-0.189616\t56.883489\t0.477000\t0.028000\n\t\n15:10:05.3\tlog_raw\tgps_raw\t\tsystem status\tnormal 2 28.200000 0 0\trobot status\t78.631600\t103.192986\t7.972500\t-0.424891\t-0.287346\t56.893109\t0.482000\t0.031000\n\t\n15:10:05.8\tlog_raw\tgps_raw\t\tsystem status\tnormal 2 28.200000 0 0\trobot status\t78.769090\t103.382837\t7.971700\t-0.375388\t-0.585063\t57.075801\t0.596000\t-0.140000\n\t\n15:10:06.3\tlog_raw\tgps_raw\t\tsystem status\tnormal 2 28.200000 0 0\trobot status\t78.909448\t103.574218\t7.971300\t-0.309070\t-0.872962\t57.206341\t0.411000\t0.106000\n\t\n15:10:06.8\tlog_raw\tgps_raw\t\tsystem status\tnormal 2 28.200000 0 0\trobot status\t79.048573\t103.764252\t7.970700\t-0.346717\t-0.685536\t57.266386\t0.469000\t0.048000\n\t\n15:10:07.3\tlog_raw\tgps_raw\t\tsystem status\tnormal 2 28.200000 0 0\trobot status\t79.190065\t103.959813\t7.968600\t-0.271988\t-0.827302\t57.383052\t0.421000\t0.098000\n\t\n15:10:07.8\tlog_raw\tgps_raw\t\tsystem status\tnormal 2 28.200000 0 0\trobot status\t79.323486\t104.150362\t7.967200\t-0.461837\t-0.577671\t57.607270\t0.456000\t0.098000\n\t\n15:10:08.3\tlog_raw\tgps_raw\t\tsystem status\tnormal 2 28.200000 0 0\trobot status\t79.461847\t104.344796\t7.963600\t-0.216859\t-0.637835\t57.778486\t0.597000\t-0.146000\n\t\n15:10:08.8\tlog_raw\tgps_raw\t\tsystem status\tnormal 2 28.200000 0 0\trobot status\t79.596985\t104.538086\t7.959700\t-0.291673\t-0.572980\t57.889616\t0.419000\t0.089000\n\t\n15:10:09.3\tlog_raw\tgps_raw\t\tsystem status\tnormal 2 28.200000 0 0\trobot status\t79.733207\t104.737724\t7.954300\t-0.515931\t-0.946723\t58.056194\t0.379000\t0.186000\n\t\n15:10:09.8\tlog_raw\tgps_raw\t\tsystem status\tnormal 2 28.100000 0 0\trobot status\t79.868217\t104.931523\t7.947200\t-0.366641\t-1.004597\t58.202165\t0.560000\t-0.106000\n\t\n15:10:10.3\tlog_raw\tgps_raw\t\tsystem status\tnormal 2 28.200000 0 0\trobot status\t80.005858\t105.129688\t7.944100\t-0.430372\t-0.969561\t58.253834\t0.470000\t0.029000\n\t\n15:10:10.8\tlog_raw\tgps_raw\t\tsystem status\tnormal 2 28.200000 0 0\trobot status\t80.142145\t105.323664\t7.940600\t-0.494415\t-0.800032\t58.276533\t0.560000\t-0.117000\n\t\n15:10:11.3\tlog_raw\tgps_raw\t\tsystem status\tnormal 2 28.200000 0 0\trobot status\t80.279182\t105.521979\t7.934000\t-0.599052\t-0.700418\t58.305150\t0.423000\t0.111000\n\t\n15:10:11.8\tlog_raw\tgps_raw\t\tsystem status\tnormal 2 28.200000 0 0\trobot status\t80.415302\t105.716328\t7.928300\t-0.475365\t-1.134146\t58.330922\t0.565000\t-0.131000\n\t\n15:10:12.3\tlog_raw\tgps_raw\t\tsystem status\tnormal 2 28.200000 0 0\trobot status\t80.551984\t105.912171\t7.925100\t-0.470450\t-0.912767\t58.371378\t0.481000\t0.029000\n\t\n15:10:12.8\tlog_raw\tgps_raw\t\tsystem status\tnormal 2 28.200000 0 0\trobot status\t80.687444\t106.107618\t7.920300\t-0.620654\t-0.556773\t58.366675\t0.488000\t0.023000\n\t\n15:10:13.3\tlog_raw\tgps_raw\t\tsystem status\tnormal 2 28.200000 0 0\trobot status\t80.827967\t106.305520\t7.915200\t-0.367035\t-0.864704\t58.361874\t0.460000\t0.022000\n\t\n15:10:13.8\tlog_raw\tgps_raw\t\tsystem status\tnormal 2 28.200000 0 0\trobot status\t80.967886\t106.503740\t7.911200\t-0.403921\t-0.711126\t58.258447\t0.497000\t0.007000\n\t\n15:10:14.3\tlog_raw\tgps_raw\t\tsystem status\tnormal 2 28.200000 0 0\trobot status\t81.103226\t106.696424\t7.907500\t-0.398812\t-0.852041\t58.114908\t0.493000\t-0.004000\n\t\n15:10:14.8\tlog_raw\tgps_raw\t\tsystem status\tnormal 2 28.200000 0 0\trobot status\t81.242532\t106.891717\t7.903500\t-0.160811\t-0.920075\t58.051028\t0.463000\t0.001000\n\t\n15:10:15.4\tlog_raw\tgps_raw\t\tsystem status\tnormal 2 28.200000 0 0\trobot status\t81.379896\t107.086416\t7.901200\t-0.292913\t-0.749500\t57.992580\t0.514000\t-0.011000\n\t\n15:10:15.9\tlog_raw\tgps_raw\t\tsystem status\tnormal 2 28.200000 0 0\trobot status\t81.518510\t107.280563\t7.898000\t-0.165432\t-0.894669\t57.901179\t0.505000\t-0.009000\n\t\n15:10:16.3\tlog_raw\tgps_raw\t\tsystem status\tnormal 2 28.200000 0 0\trobot status\t81.656725\t107.472667\t7.896000\t-0.032483\t-0.793907\t57.815540\t0.483000\t0.002000\n\t\n15:10:16.9\tlog_raw\tgps_raw\t\tsystem status\tnormal 2 28.200000 0 0\trobot status\t81.798207\t107.668605\t7.894300\t-0.086703\t-0.852911\t57.686714\t0.497000\t-0.004000\n\t\n15:10:17.4\tlog_raw\tgps_raw\t\tsystem status\tnormal 2 28.200000 0 0\trobot status\t81.938514\t107.858326\t7.891500\t0.205832\t-0.594837\t57.590581\t0.504000\t-0.005000\n\t\n15:10:17.8\tlog_raw\tgps_raw\t\tsystem status\tnormal 2 28.200000 0 0\trobot status\t82.082717\t108.052930\t7.888000\t0.227829\t-0.778987\t57.523090\t0.501000\t-0.004000\n\t\n15:10:18.4\tlog_raw\tgps_raw\t\tsystem status\tnormal 2 28.200000 0 0\trobot status\t82.220659\t108.243380\t7.886800\t-0.039639\t-0.495216\t57.411198\t0.491000\t-0.003000\n\t\n15:10:18.9\tlog_raw\tgps_raw\t\tsystem status\tnormal 2 28.200000 0 0\trobot status\t82.364330\t108.436733\t7.884600\t0.258471\t-0.535635\t57.340567\t0.495000\t-0.003000\n\t\n15:10:19.4\tlog_raw\tgps_raw\t\tsystem status\tnormal 2 28.200000 0 0\trobot status\t82.499849\t108.623961\t7.884800\t0.046509\t-0.357204\t57.314348\t0.485000\t-0.003000\n\t\n15:10:19.9\tlog_raw\tgps_raw\t\tsystem status\tnormal 2 28.200000 0 0\trobot status\t82.642105\t108.823260\t7.883300\t-0.301239\t-0.225368\t57.128616\t0.503000\t-0.013000\n\t\n15:10:20.4\tlog_raw\tgps_raw\t\tsystem status\tnormal 2 28.200000 0 0\trobot status\t82.779109\t109.009306\t7.883300\t-0.331380\t-0.090803\t56.974713\t0.486000\t-0.005000\n\t\n15:10:20.9\tlog_raw\tgps_raw\t\tsystem status\tnormal 2 28.200000 0 0\trobot status\t82.918557\t109.199561\t7.887900\t-0.546059\t-0.226655\t56.895526\t0.488000\t-0.007000\n\t\n15:10:21.4\tlog_raw\tgps_raw\t\tsystem status\tnormal 2 28.200000 0 0\trobot status\t83.062361\t109.392647\t7.886400\t-0.361209\t-0.499872\t56.770094\t0.495000\t0.002000\n\t\n15:10:21.9\tlog_raw\tgps_raw\t\tsystem status\tnormal 2 28.200000 0 0\trobot status\t83.205200\t109.584098\t7.884100\t-0.301466\t-0.608732\t56.618339\t0.501000\t-0.013000\n\t\n15:10:22.4\tlog_raw\tgps_raw\t#INSPVAXA,USB3,0,50.0,FINESTEERING,2107,281440.400,02000000,471d,15824;INS_ALIGNMENT_COMPLETE,INS_RTKFIXED,37.37111948466,126.72177620543,7.8818,22.3000,0.3548,0.3148,0.0036,-0.259281902,-0.804731473,33.477876522,0.4069,0.2838,0.5238,0.1105,0.0914,0.0781,0.2627,0.2373,5.1917,0f000001,0*1022e28e\n\tsystem status\tnormal 2 28.200000 0 0\trobot status\t83.361126\t109.795335\t7.881800\t-0.259282\t-0.804731\t56.522123\t0.497000\t-0.006000\n\t\n15:10:22.9\tlog_raw\tgps_raw\t\tsystem status\tnormal 2 28.200000 0 0\trobot status\t83.489703\t109.964418\t7.878900\t0.059859\t-0.788033\t56.364114\t0.503000\t-0.013000\n\t\n15:10:23.4\tlog_raw\tgps_raw\t\tsystem status\tnormal 2 28.200000 0 0\trobot status\t83.634114\t110.156316\t7.877000\t0.169319\t-0.664888\t56.240043\t0.501000\t0.003000\n\t\n15:10:23.9\tlog_raw\tgps_raw\t\tsystem status\tnormal 2 28.200000 0 0\trobot status\t83.774521\t110.346974\t7.875700\t-0.202590\t-0.796526\t56.384423\t0.596000\t-0.146000\n\t\n15:10:24.4\tlog_raw\tgps_raw\t\tsystem status\tnormal 2 28.200000 0 0\trobot status\t83.917633\t110.537744\t7.875000\t0.111906\t-0.680142\t56.728808\t0.427000\t0.097000\n\t\n15:10:24.9\tlog_raw\tgps_raw\t\tsystem status\tnormal 2 28.200000 0 0\trobot status\t84.056300\t110.728326\t7.873700\t0.112114\t-0.438575\t57.002476\t0.466000\t0.046000\n\t\n15:10:25.4\tlog_raw\tgps_raw\t\tsystem status\tnormal 2 28.200000 0 0\trobot status\t84.195099\t110.921753\t7.873200\t0.086569\t-0.625307\t57.243757\t0.486000\t0.013000\n\t\n15:10:25.9\tlog_raw\tgps_raw\t\tsystem status\tnormal 2 28.200000 0 0\trobot status\t84.331934\t111.117005\t7.873500\t-0.155630\t-0.288073\t57.475141\t0.431000\t0.102000\n\t\n15:10:26.4\tlog_raw\tgps_raw\t\tsystem status\tnormal 2 28.100000 0 0\trobot status\t84.466995\t111.306754\t7.872400\t0.030142\t-0.009179\t57.782380\t0.412000\t0.150000\n\t\n15:10:26.9\tlog_raw\tgps_raw\t\tsystem status\tnormal 2 28.200000 0 0\trobot status\t84.602535\t111.498596\t7.872600\t-0.011316\t-0.006006\t57.822911\t0.540000\t-0.092000\n\t\n15:10:27.4\tlog_raw\tgps_raw\t\tsystem status\tnormal 2 28.200000 0 0\trobot status\t84.739704\t111.693841\t7.873700\t-0.009358\t-0.049625\t57.765796\t0.504000\t-0.021000\n\t\n15:10:27.9\tlog_raw\tgps_raw\t\tsystem status\tnormal 2 28.200000 0 0\trobot status\t84.873943\t111.883613\t7.874200\t0.023205\t-0.261764\t57.685405\t0.504000\t-0.015000\n\t\n15:10:28.4\tlog_raw\tgps_raw\t\tsystem status\tnormal 2 28.200000 0 0\trobot status\t85.012193\t112.079946\t7.875100\t-0.115125\t-0.378789\t57.618527\t0.493000\t-0.014000\n\t\n15:10:28.9\tlog_raw\tgps_raw\t\tsystem status\tnormal 2 28.200000 0 0\trobot status\t85.148561\t112.268411\t7.877800\t-0.022533\t-0.476139\t57.384668\t0.498000\t-0.012000\n\t\n15:10:29.4\tlog_raw\tgps_raw\t\tsystem status\tnormal 2 28.200000 0 0\trobot status\t85.287319\t112.458849\t7.877800\t0.032470\t-0.280697\t57.133854\t0.497000\t-0.019000\n\t\n15:10:29.9\tlog_raw\tgps_raw\t\tsystem status\tnormal 2 28.200000 0 0\trobot status\t85.424695\t112.645727\t7.877600\t-0.032757\t-0.430103\t56.874549\t0.492000\t-0.021000\n\t\n15:10:30.4\tlog_raw\tgps_raw\t\tsystem status\tnormal 2 28.200000 0 0\trobot status\t85.569128\t112.841634\t7.876700\t0.045968\t-0.560552\t56.600652\t0.491000\t-0.026000\n\t\n15:10:30.9\tlog_raw\tgps_raw\t\tsystem status\tnormal 2 28.200000 0 0\trobot status\t85.716386\t113.040442\t7.873200\t0.039345\t-0.348564\t56.298044\t0.499000\t-0.029000\n\t\n15:10:31.4\tlog_raw\tgps_raw\t\tsystem status\tnormal 2 28.200000 0 0\trobot status\t85.860562\t113.228525\t7.872900\t0.257444\t-0.144228\t55.935097\t0.502000\t-0.005000\n\t\n15:10:31.9\tlog_raw\tgps_raw\t\tsystem status\tnormal 2 28.200000 0 0\trobot status\t86.011614\t113.421914\t7.874800\t0.290012\t-0.182649\t55.562325\t0.493000\t-0.024000\n\t\n15:10:32.4\tlog_raw\tgps_raw\t\tsystem status\tnormal 2 28.200000 0 0\trobot status\t86.159994\t113.612818\t7.876100\t0.053591\t-0.222503\t55.045035\t0.513000\t-0.026000\n\t\n15:10:32.9\tlog_raw\tgps_raw\t\tsystem status\tnormal 2 28.100000 0 0\trobot status\t86.310870\t113.799257\t7.877200\t0.232244\t-0.275979\t54.308223\t0.503000\t-0.029000\n\t\n15:10:33.4\tlog_raw\tgps_raw\t#INSPVAXA,USB3,0,47.0,FINESTEERING,2107,281451.400,02000000,471d,15824;INS_ALIGNMENT_COMPLETE,INS_RTKFIXED,37.37115737794,126.72181140198,7.8793,22.3000,0.3546,0.3544,0.0026,0.301499965,-0.418827265,36.616680382,0.4121,0.2951,0.5421,0.1113,0.0929,0.0791,0.2623,0.2370,5.2056,0f000001,0*452f9763\n\tsystem status\tnormal 2 28.100000 0 0\trobot status\t86.478779\t114.000875\t7.879300\t0.301500\t-0.418827\t53.383320\t0.403000\t-0.153000\n\t\n15:10:33.9\tlog_raw\tgps_raw\t\tsystem status\tnormal 2 28.100000 0 0\trobot status\t86.619422\t114.162496\t7.881200\t0.338868\t-0.472813\t52.461615\t0.571000\t0.109000\n\t\n15:10:34.4\tlog_raw\tgps_raw\t#INSPVAXA,USB3,0,44.5,FINESTEERING,2107,281452.400,02000000,471d,15824;INS_ALIGNMENT_COMPLETE,INS_RTKFIXED,37.37116058120,126.72181495507,7.8824,
